vi "newImageStringEvent.vi"(8 "error in (no error)":errorcluster, 10 "ImageString":string, 11 "ImageStreamViewer in":refnum<class "ImageStreamViewer.lvclass">) -> (0 "error out":errorcluster, 3 "ImageStreamViewer out":refnum<class "ImageStreamViewer.lvclass">)   [LabVIEW 2009, in "Views.lvlib" / "Camera.lvlib" / "ImageStreamViewer.lvclass"]
uses:
  ImageStreamViewer.lvclass
  ImageStreamViewer.lvclass/ImageStreamViewer.ctl
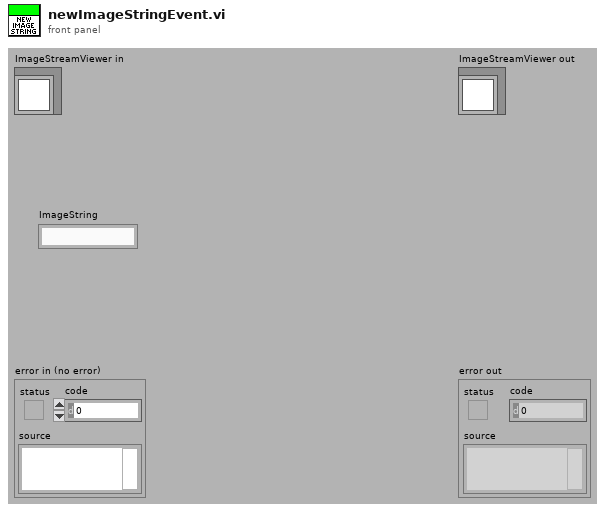
[diagram p1: front panel]
types:
  T1 = typedef "IMAQ Image.ctl" = refnum<image>
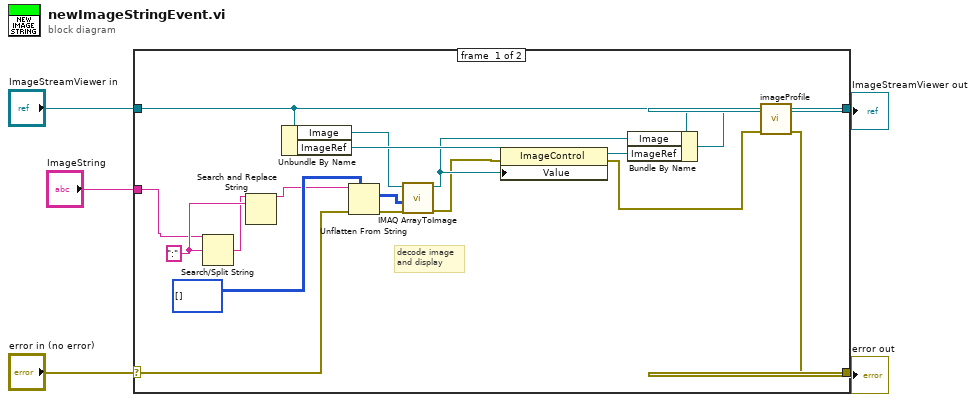
[diagram p0: block diagram]
diagram:
  n1 = case shown="No Error" "error in (no error)" {
    selector: "error in (no error)" -> [w23 w25]
    tunnel: [w11 w25] -> w4
    tunnel: [w14 w24] -> w2
    tunnel: "ImageStreamViewer in" -> [w20 w24]
    tunnel: "ImageString" -> [w16 _]
    frame #0 {
      w18 = ":"
      # "decode image\nand display"
      n2 = Search/Split String(string=w16, search string/char (-)=w18) -> (match + rest of string=w17:string)  [unwired: 1 in, 2 out]
      n3 = Search and Replace String(input string=w17, search string=w18) -> (result string=w15:string)  [unwired: 6 in, 3 out]
      n4 = Unbundle By Name(w20) -> ("Image"=w7:T1, "ImageRef"=w22:refnum<vi>)
      n5 = Unflatten From String(type=u16[][] [] ("Image data"), binary string=w15, error in (no error)=w23) -> (value=w6:u16[][], error out=w10:errorcluster)  [unwired: 2 in, 1 out]
      n6 = call "IMAQ ArrayToImage"("error in (no error)"=w10, "Image Pixels (I16)"=w6, "Image"=w7) -> ("error out"=w8:errorcluster, "Image Out"=w9:T1)  [unwired: 7 in]
      n7 = property class="ImageControl"(reference=w22, error in=w8, "Value"=w9) -> (reference out=w21:refnum<vi>, error out=w12:errorcluster)
      n8 = Bundle By Name(cluster=w20, "Image"=w9, "ImageRef"=w21) -> (w13:refnum<class "ImageStreamViewer.lvclass">)
      n9 = call "imageProfile.vi"("error in (no error)"=w12, "ImageStreamViewer in"=w13) -> ("error out"=w11:errorcluster, "ImageStreamViewer out"=w14:refnum<class "ImageStreamViewer.lvclass">)  [unwired: 8 in]
    }
    frame #1 {
    }
  }
  "error out" <- w4
  "ImageStreamViewer out" <- w2
